vi "Comp_4_Elements.vi"(0 "CompVal":u16, 5 "Array":u16[](array[numeric])) -> (4 "result":bool)   [LabVIEW 2016]
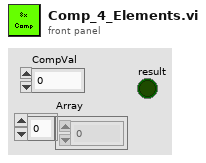
[diagram p1: front panel]
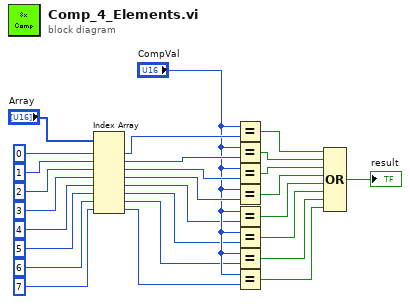
[diagram p0: block diagram]
diagram:
  n1 = Index Array(array="Array", index #1=0 ("index"), index #2=1 ("index"), index #3=2 ("index"), index #4=3 ("index"), index #5=4 ("index"), index #6=5 ("index"), index #7=6 ("index"), index #8=7 ("index")) -> (element #1=w21:u16, element #2=w20:u16, element #3=w19:u16, element #4=w18:u16, element #5=w12:u16, element #6=w11:u16, element #7=w10:u16, element #8=w9:u16)
  n2 = Equal?(x="CompVal", y=w21) -> (x = y?=w24:bool)
  n3 = Equal?(x="CompVal", y=w20) -> (x = y?=w25:bool)
  n4 = Equal?(x="CompVal", y=w19) -> (x = y?=w26:bool)
  n5 = Equal?(x="CompVal", y=w18) -> (x = y?=w27:bool)
  n6 = Equal?(x="CompVal", y=w12) -> (x = y?=w8:bool)
  n7 = Equal?(x="CompVal", y=w11) -> (x = y?=w7:bool)
  n8 = Equal?(x="CompVal", y=w10) -> (x = y?=w6:bool)
  n9 = Equal?(x="CompVal", y=w9) -> (x = y?=w5:bool)
  n10 = Compound Arithmetic op=OR(w24, w25, w26, w27, w8, w7, w6, w5) -> (→"result":bool)
